vi "LV-TOML Test Marshall-Unmarshall.vi"() -> ()   [LabVIEW 2020]
uses:
  <vilib>/LabVIEW Open Source Project/OpenSerializer/Serializer/Serializer.lvclass
  source/Serializer.LV-TOML.lvclass
  C:/Program Files (x86)/National Instruments/LabVIEW 2020/vi.lib/LabVIEW Open Source Project/OpenSerializer/Serializer/Serializer.lvclass
  LV-TOML Test Data_Cluster.ctl
panel:
  out "error out":errorcluster
  out "Pass?":bool
  out "Data Cluster out":T1={"Top-Level Cluster"={"Boolean"=FALSE, "String"="", "Path"="", "Numeric"=0.0, "Enum"=enum."Item0", "Array"=[], "Sub-Cluster"={"Numeric"=4.0, "Boolean"=FALSE, "String"=""}, "Multi-Line String"="Another test string"}} {"Top-Level Cluster"."Numeric" format="%#_10g"}
  out "TOML String":string
  in  "Data Cluster in":T1={"Top-Level Cluster"={"Boolean"=FALSE, "String"="Another test string", "Path"="C:\\Windows", "Numeric"=3.141592654, "Enum"=enum."Item0", "Array"=[0.0, 1.0, 2.0, 3.0, 4.0, 5.0, 6.0], "Sub-Cluster"={"Numeric"=4.0, "Boolean"=TRUE, "String"="Test String Here"}, "Multi-Line String"="Another test string\nLine2\nLine3"}} {"Top-Level Cluster"."Numeric" format="%#_10g"}
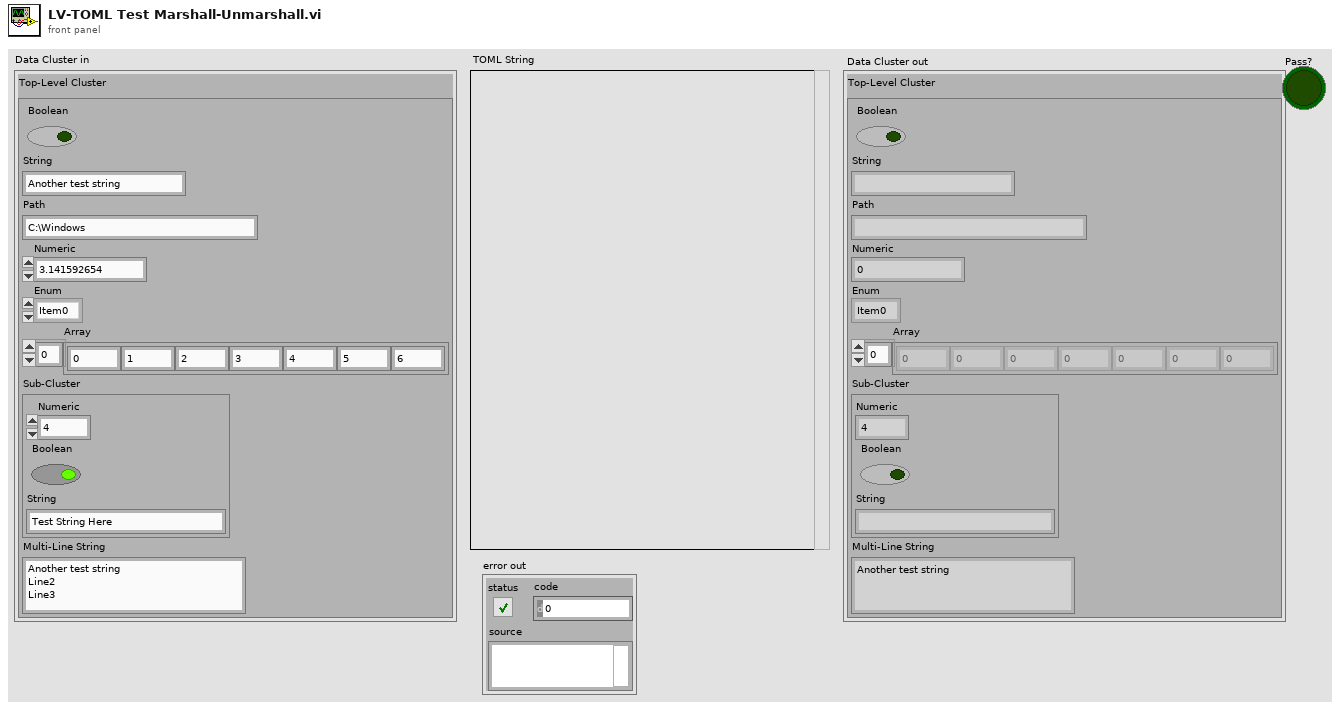
[diagram p1: front panel]
types:
  T1 = typedef "LV-TOML Test Data_Cluster.ctl" = cluster{"Top-Level Cluster":cluster{"Boolean":bool, "String":string, "Path":string, "Numeric":dbl, "Enum":enum16{"Item0", "Item1"}, "Array":dbl[], "Sub-Cluster":cluster{"Numeric":dbl, "Boolean":bool, "String":string}, "Multi-Line String":string}}
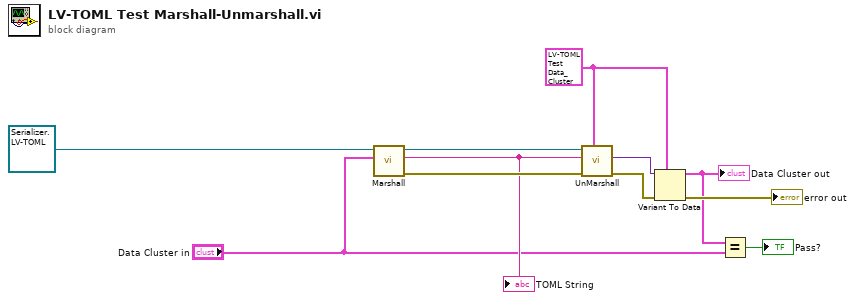
[diagram p0: block diagram]
diagram:
  w6 = T1 {"Top-Level Cluster"={"Boolean"=FALSE, "String"="", "Path"="", "Numeric"=0.0, "Enum"=enum."Item0", "Array"=[], "Sub-Cluster"={"Numeric"=4.0, "Boolean"=FALSE, "String"=""}, "Multi-Line String"="Another test string"}} ("Cluster")
  n1 = call <vilib>:"Marshall.vi"("Variant"="Data Cluster in", "Serializer in"=refnum<class "Serializer.LV-TOML.lvclass"> refnum ("OpenSerializer.erdosmiller-TOML.lvlib:Serializer.erdosmiller-TOML.lvclass")) -> ("error out"=w11:errorcluster, "String"=w9:string, "Serializer out"=w10:refnum<class "Serializer.LV-TOML.lvclass">)  [unwired: 7 in]
  "TOML String" <- w9
  n2 = call <vilib>:"UnMarshall.vi"("Type"=w6, "error in (no error)"=w11, "String"=w9, "Serializer in"=w10) -> ("error out"=w8:errorcluster, "Variant"=w7:variant)  [unwired: 5 in, 1 out]
  n3 = Variant To Data(error in=w8, type=w6, Variant=w7) -> (data=w1:T1, error out=→"error out":errorcluster)
  "Data Cluster out" <- w1
  n4 = Equal?(x=w1, y="Data Cluster in") -> (x = y?=→"Pass?":bool)
